vi "Actor Last Ack.vi"(10 "Nested Actor":refnum<class "Actor.lvclass">, 11 "Dev Actor in":refnum<class "Dev Actor.lvclass">) -> (3 "Dev Actor out":refnum<class "Dev Actor.lvclass">)   [LabVIEW 2021, in "Dev Actor.lvlib" / "Dev Actor.lvclass"]
uses:
  Dev Actor.lvclass
  <vilib>/jettl/jettl/jettl/Actor/Actor.lvclass
  Dev Actor.lvclass/Dev Actor.ctl
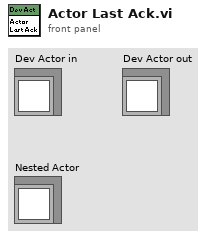
[diagram p1: front panel]
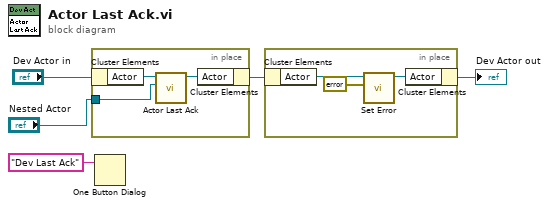
[diagram p0: block diagram]
diagram:
  n1 = in-place {
    in-place-border: "Nested Actor" -> [w8]
    n2 = in-place-cluster #1("Dev Actor in") -> ("Actor"=w6:refnum<class "Actor.lvclass">)
    n3 = call-dynamic "Actor Last Ack.vi"("Nested Actor"=w8, "Actor Last Ack in"=w6) -> ("Actor Last Ack out"=w7:refnum<class "Actor.lvclass">)  [unwired: 9 in]
    n4 = in-place-cluster #1("Actor"=w7) -> (w2:refnum<class "Dev Actor.lvclass">)
  }
  n5 = One Button Dialog(message="Dev Last Ack") -> ()  [unwired: 1 in, 1 out]
  n6 = in-place {
    n7 = in-place-cluster #2(w2) -> ("Actor"=w11:refnum<class "Actor.lvclass">)
    n8 = call-dynamic "Set Error.vi"("Error"=errorcluster {"status"=FALSE, "code"=0, "source"=""}, "Actor in"=w11) -> ("Actor out"=w10:refnum<class "Actor.lvclass">)  [unwired: 9 in]
    n9 = in-place-cluster #2("Actor"=w10) -> (→"Dev Actor out":refnum<class "Dev Actor.lvclass">)
  }
